vi "UDP Transmit.vi"(8 "error in (no error)":errorcluster, 9 "Tx":T1, 10 "Transfers":refnum<class "Transfer.lvclass">[](array[class]), 11 "UDP Transceiver in":refnum<class "UDP Transceiver.lvclass">) -> (0 "error out":errorcluster, 3 "UDP Transceiver out":refnum<class "UDP Transceiver.lvclass">)   [LabVIEW 2017, in "UDP.lvlib" / "UDP Transceiver.lvclass"]
uses:
  UDP Transceiver.lvclass
  Builds/Data Sharing Framework/Current/Data Sharing Framework Core/DSF Core.lvlibp/Engine/Classes/Transfer/Transfer.lvclass
  Transfer Group Tx Parameters.ctl
  Transfer Tx Parameters.ctl
  UDP Transceiver.lvclass/UDP Transceiver.ctl
  Builds/Data Sharing Framework/Current/Data Sharing Framework Core/DSF Core.lvlibp/Engine/Classes/Buffer/Read Buffer 1D U8.vi
  Builds/Data Sharing Framework/Current/Data Sharing Framework Core/DSF Core.lvlibp/Engine/Classes/Buffer/Buffer.lvclass
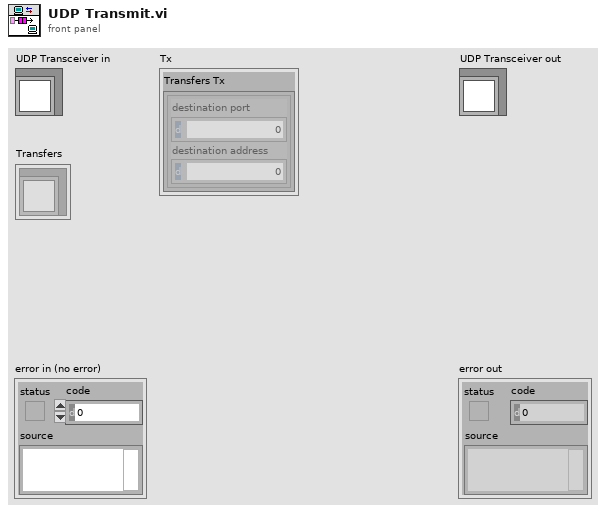
[diagram p1: front panel]
types:
  T1 = typedef "UDP.lvlib/UDP Transceiver.lvclass/Transfer Group Tx Parameters.ctl" = cluster{"Transfers Tx":T2[]}
  T2 = typedef "UDP.lvlib/UDP Transceiver.lvclass/Transfer Tx Parameters.ctl" = cluster{"destination port":u16, "destination address":u32}
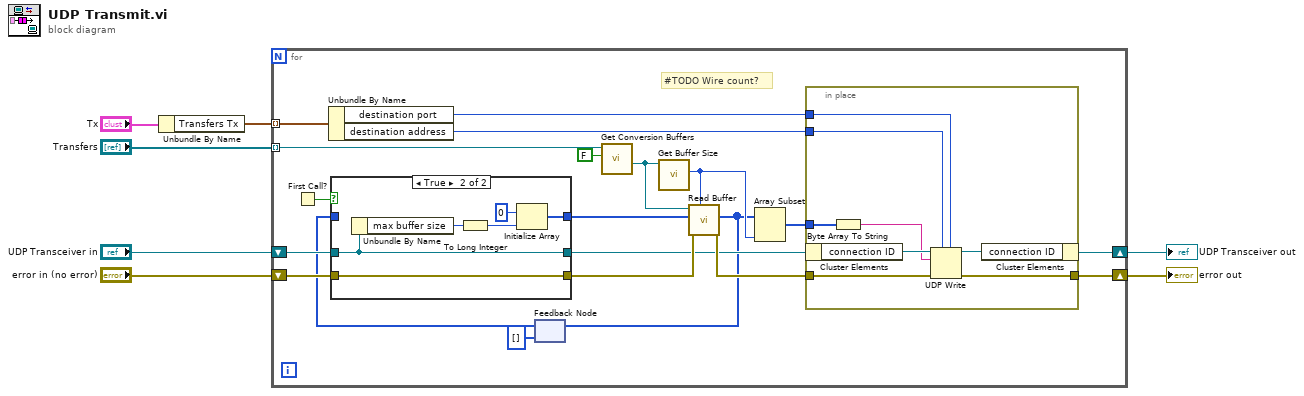
[diagram p0: block diagram]
diagram:
  n1 = Unbundle By Name("Tx") -> ("Transfers Tx"=w7:T2[])
  n2 = for {
    tunnel: "Transfers" -> [w14] mode=indexing
    tunnel: w7 -> [w15] mode=indexing
    shift-right: [w27] -> w4
    shift-left: "error in (no error)" -> [w23]
    shift-right: [w26] -> w3
    shift-left: "UDP Transceiver in" -> [w17]
    # "#TODO Wire count?"
    n3 = First Call?() -> (First Call?: T/F=w21:bool)
    n4 = Unbundle By Name(w15) -> ("destination port"=w25:u16, "destination address"=w9:u32)
    n5 = feedback #1(u8[] [] ("buffer out")) -> (w16:u8[])
    n6 = case shown="True" w21 {
      tunnel: w17 -> [w29 w35]
      tunnel: w23 -> [w30 w36]
      tunnel: [w30 w36] -> w22
      tunnel: [w29 w35] -> w18
      tunnel: w16 -> [w28 _]
      tunnel: [w28 w32] -> w11
      frame False {
      }
      frame True {
        n7 = Unbundle By Name(w35) -> ("max buffer size"=w34:u64)
        n8 = To Long Integer(number=w34) -> (32bit integer=w31:i32)
        n9 = Initialize Array(u8 0 ("element"), w31) -> (w32:u8[])
      }
    }
    n10 = call "Get Conversion Buffers.vi"("inline?"=FALSE, "Transfer in"=w14) -> ("converted Buffer"=w12:refnum<class "Buffer.lvclass">)  [unwired: 6 in, 3 out]
    n11 = call "Get Buffer Size.vi"("Buffer in"=w12) -> ("buffer size"=w13:u64)  [unwired: 9 in, 1 out]
    n12 = call-poly "Read Buffer.vi"("count (-1: rest)"=w13, "error in (no error)"=w22, "dst array in"=w11, "Buffer in"=w12) -> ("error out"=w24:errorcluster, "dst array out"=w10:u8[])  [unwired: 4 in, 2 out]
    n13 = feedback-in #1(w10) -> ()
    n14 = Array Subset(array=w10, length=w13) -> (w20:u8[])  [unwired: 1 in]
    n15 = in-place {
      in-place-border: w24 -> [w44]
      in-place-border: [w41] -> w27
      in-place-border: w9 -> [w40]
      in-place-border: w25 -> [w39]
      in-place-border: w20 -> [w38]
      n16 = in-place-cluster #2(w18) -> ("connection ID"=w43:refnum<k16>)
      n17 = Byte Array To String(unsigned byte array=w38) -> (string=w37:string)
      n18 = UDP Write(address=w40, port or service name=w39, connection ID=w43, data in=w37, 8:w44) -> (error out=w41:errorcluster, 3:w42:refnum<k16>)  [unwired: 1 in]
      n19 = in-place-cluster #2("connection ID"=w42) -> (w26:refnum<class "UDP Transceiver.lvclass">)
    }
  }
  "error out" <- w4
  "UDP Transceiver out" <- w3
